vi "Write Delta Ref.vi"(8 "error in (no error)":errorcluster, 10 "Delta Ref":refnum<vi>, 11 "Analyze Results Beam Deviation in":refnum<class "Analyze Results Beam Deviation.lvclass">) -> (0 "error out":errorcluster, 3 "Analyze Results Beam Deviation out":refnum<class "Analyze Results Beam Deviation.lvclass">)   [LabVIEW 2014, in "Analyze Results Beam Deviation.lvclass"]
uses:
  Analyze Results Beam Deviation.lvclass
  Analyze Results Beam Deviation.lvclass/Analyze Results Beam Deviation.ctl
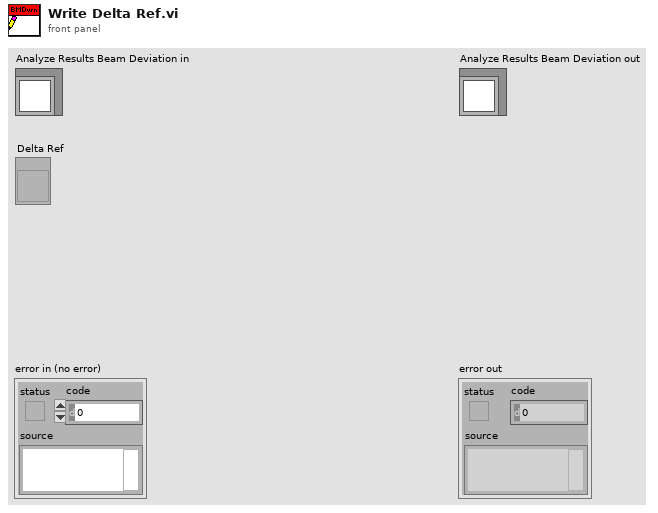
[diagram p1: front panel]
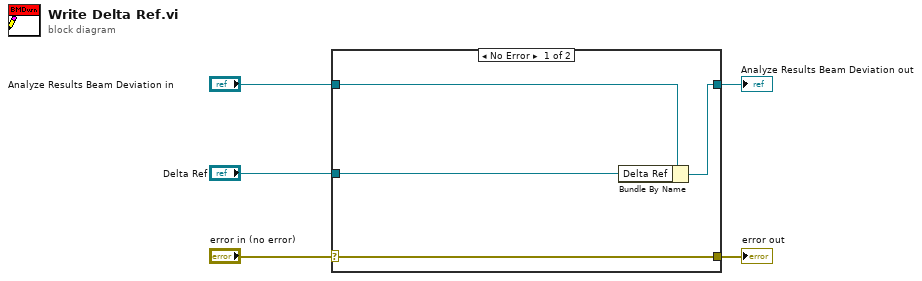
[diagram p0: block diagram]
diagram:
  n1 = case shown="No Error" "error in (no error)" {
    selector: "error in (no error)" -> [w9 w10]
    tunnel: [w9 w10] -> w4
    tunnel: [w7 w11] -> w2
    tunnel: "Analyze Results Beam Deviation in" -> [w8 w11]
    tunnel: "Delta Ref" -> [w6 _]
    frame No Error {
      n2 = Bundle By Name(cluster=w8, "Delta Ref"=w6) -> (w7:refnum<class "Analyze Results Beam Deviation.lvclass">)
    }
    frame Error {
    }
  }
  "error out" <- w4
  "Analyze Results Beam Deviation out" <- w2
